vi "main.vi"() -> ()   [LabVIEW 2009]
uses:
  <vilib>/Instr/_visa.llb/VISA Configure Serial Port (Instr).vi
panel:
  in  "delay before read (ms)":u32=500 caption="读取前延时(ms)"
  in  "flow control":u16(ring) caption="流程控制" items=["无"=0, "XON/XOFF"=1, "RTS/CTS"=2, "DTR/DSR"=4]
  in  "stop bits":u16(ring)=10 caption="停止位" items=["1.0"=10, "1.5"=15, "2.0"=20]
  in  "parity":u16(ring) caption="奇偶" items=["无", "奇", "偶", "标记", "空格"]
  in  "data bits":u16=8 caption="数据比特" min=5 max=8 step=1
  in  "read":bool=TRUE caption="读取"
  in  "write":bool=TRUE caption="写入"
  out "bytes read":u32 caption="读取的字节"
  out "read string":string caption="读取字符串"
  in  "VISA resource name":refnum<visa-resource-name>="COM1" caption="VISA资源名称"
  in  "baud rate":u32=9600 caption="波特率"
  in  "Spoken Text":string
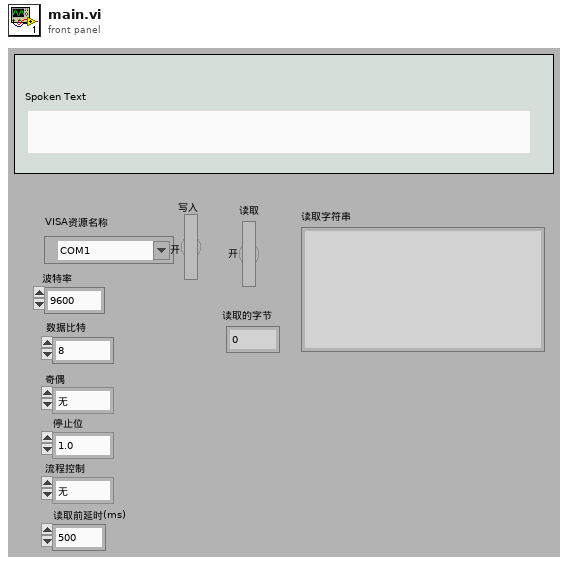
[diagram p1: front panel]
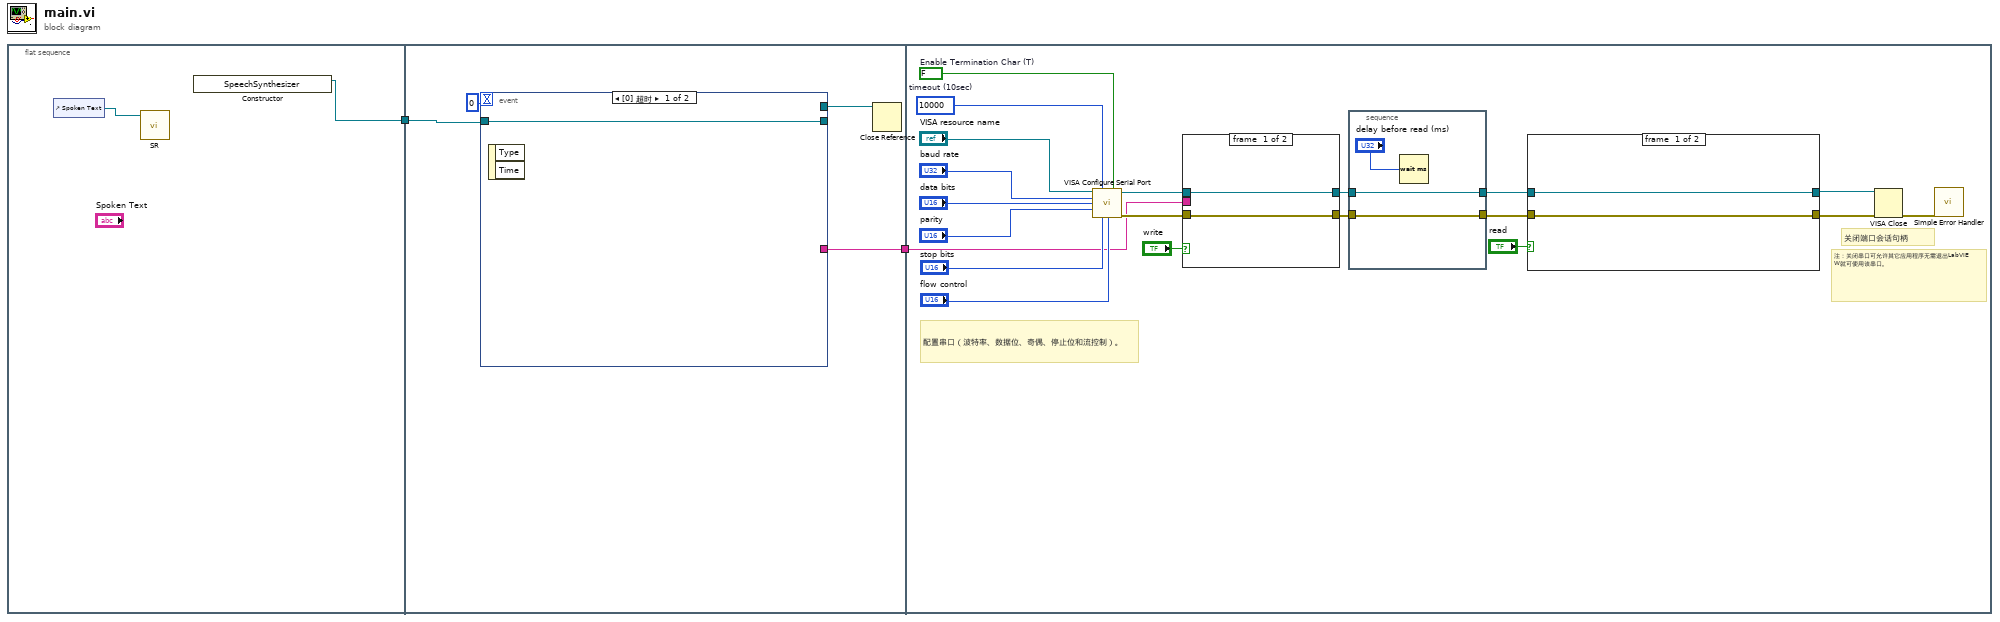
[diagram p0: block diagram]
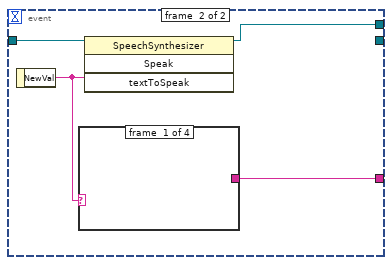
[diagram p2: hidden frame]
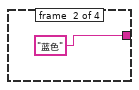
[diagram p3: hidden frame]
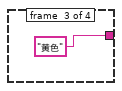
[diagram p4: hidden frame]
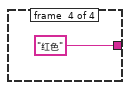
[diagram p5: hidden frame]
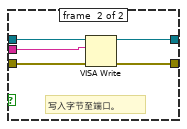
[diagram p6: hidden frame]
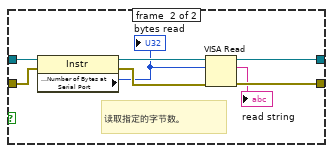
[diagram p7: hidden frame]
diagram:
  n1 = flat-sequence {
    tunnel: [w4] -> w2
    tunnel: w2 -> [w8]
    tunnel: [w6] -> w1
    tunnel: w1 -> [w17]
    frame #0 {
      n2 = control-ref of="Spoken Text"() -> (w3:refnum<vi>)
      n3 = call "SR.vi"("Spoken text box"=w3) -> ()  [unwired: 6 in, 1 out]
      n4 = constructor class="SpeechSynthesizer"() -> (reference out=w4:refnum<k24>)  [unwired: 3 in, 2 out]
    }
    frame #1 {
      n5 = event shown="[0] 超时" {
        selector: _ -> [_ _]
        dyn-events: _ -> [_ _]
        timeout: 0 -> [_ _]
        tunnel: w8 -> [w9 w13]
        tunnel: [w9 _] -> _
        tunnel: [_ w11] -> w7
        tunnel: [_ w10] -> w6
        event #0 {
          n6 = event-data() -> ()  [unwired: 1 in, 2 out]
        }
        event #1 {
          n7 = event-data() -> ("NewVal"=w12:string)  [unwired: 1 in]
          n8 = case shown="\"红色\"" w12 {
            tunnel: [_ "蓝色" "黄色" "红色"] -> w10
            frame #0 {
            }
            frame #1 {
            }
            frame #2 {
            }
            frame #3 {
            }
          }
          n9 = invoke class="SpeechSynthesizer" method="Speak"(reference=w13, "textToSpeak"=w12) -> (reference out=w11:refnum<k24>)  [unwired: 2 in, 3 out]
        }
      }
      n10 = Close Reference(reference=w7) -> ()  [unwired: 1 in, 1 out]
    }
    frame #2 {
      w26 = FALSE  # Enable Termination Char (T)
      w27 = u32 10000  # timeout (10sec)
      # "注：关闭串口可允许其它应用程序无需退出LabVIEW就可使用该串口。"
      # "配置串口（波特率、数据位、奇偶、停止位和流控制）。"
      # "关闭端口会话句柄"
      n11 = call-poly "VISA Configure Serial Port"("VISA resource name"="VISA resource name", "timeout (10sec)"=w27, "Enable Termination\nChar (T)"=w26, "baud rate (9600)"="baud rate", "data bits (8)"="data bits", "parity (0:none)"="parity", "stop bits (10: 1 bit)"="stop bits", "flow control (0:none)"="flow control") -> ("VISA resource name out"=w32:refnum<visa-resource-name>, "error out"=w33:errorcluster)  [unwired: 1 in, 5 out]
      n12 = case shown="真" "write" {
        tunnel: [w41 w46] -> w21
        tunnel: w32 -> [w40 w45]
        tunnel: w33 -> [w41 w44]
        tunnel: [w40 w43] -> w19
        tunnel: w17 -> [_ w42]
        frame #0 {
        }
        frame #1 {
          # "写入字节至端口。"
          n13 = VISA Write(VISA resource name=w45, write buffer=w42, error in (no error)=w44) -> (VISA resource name out=w43:refnum<visa-resource-name>, error out=w46:errorcluster)  [unwired: 1 out]
        }
      }
      n14 = stacked-sequence {
        tunnel: w21 -> [w39]
        tunnel: [w39] -> w20
        tunnel: w19 -> [w38]
        tunnel: [w38] -> w18
        frame #0 {
          n15 = Wait (ms)(milliseconds to wait="delay before read (ms)") -> ()  [unwired: 1 out]
        }
      }
      n16 = case shown="真" "read" {
        tunnel: w20 -> [w48 w52]
        tunnel: [w48 w56] -> w31
        tunnel: [w47 w55] -> w30
        tunnel: w18 -> [w47 w54]
        frame #0 {
        }
        frame #1 {
          # "读取指定的字节数。"
          n17 = property class="Instr"(reference=w54, error in=w52) -> (reference out=w53:refnum<visa-resource-name>, error out=w51:errorcluster, "Serial Settings:Number of Bytes at Serial Port"=w49:u32)
          "bytes read" <- w49
          n18 = VISA Read(VISA resource name=w53, byte count=w49, error in (no error)=w51) -> (VISA resource name out=w55:refnum<visa-resource-name>, read buffer=→"read string":string, error out=w56:errorcluster)  [unwired: 1 out]
        }
      }
      n19 = VISA Close(VISA resource name=w30, error in (no error)=w31) -> (error out=w29:errorcluster)
      n20 = call <vilib>:"Simple Error Handler.vi"("error in (no error)"=w29) -> ()  [unwired: 1 in, 8 out]
    }
  }
